vi "Add System.vi"(8 "error in (no error)":errorcluster, 11 "Manager in":refnum<class "Manager.lvclass">) -> (0 "error out":errorcluster, 3 "Manager out":refnum<class "Manager.lvclass">)   [LabVIEW 2013, in "Manager.lvlib" / "Manager.lvclass"]
uses:
  Manager.lvclass
  PluginInterface/Actor Framework.lvlibp/Actor/Actor.lvclass
  Manager Messages/Update SubPanel Msg/Update SubPanel Msg.lvclass
  <vilib>/Utility/LVLibp/NI_PackedLibraryUtility.lvlib
  PluginInterface/PluginInterface.lvlibp/PluginInterfaceClass/PluginInterface.lvclass
  PluginInterface/Actor Framework.lvlibp/Message Enqueuer/Message Enqueuer.lvclass
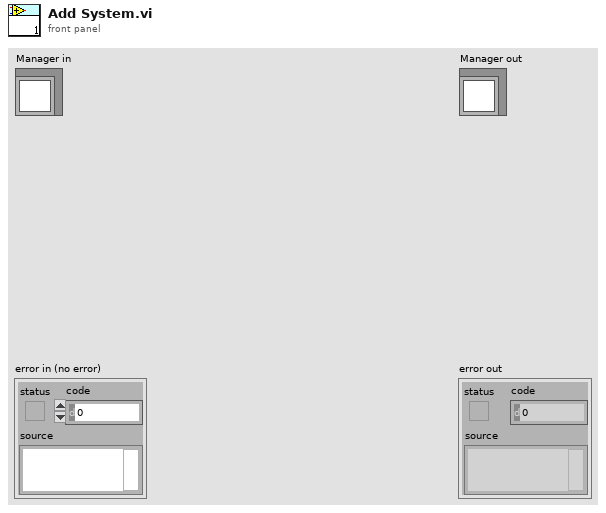
[diagram p1: front panel]
types:
  T1 = cluster{string, "Caller-To-Actor Enqueuer":refnum<class "Message Enqueuer.lvclass">}
  T2 = cluster{"Name":string, "Plugins":cluster{"Name":string, "Plugin":refnum<class "Message Enqueuer.lvclass">}[]}[]
  T3 = cluster{"Name":string, cluster{string, "Caller-To-Actor Enqueuer":refnum<class "Message Enqueuer.lvclass">}[]}
  T4 = cluster{"Name":string, "Plugins":cluster{"Name":string, "Caller-To-Actor Enqueuer":refnum<class "Message Enqueuer.lvclass">}[]}[]
  T5 = cluster{"Name":string, refnum<class "Message Enqueuer.lvclass">[]}
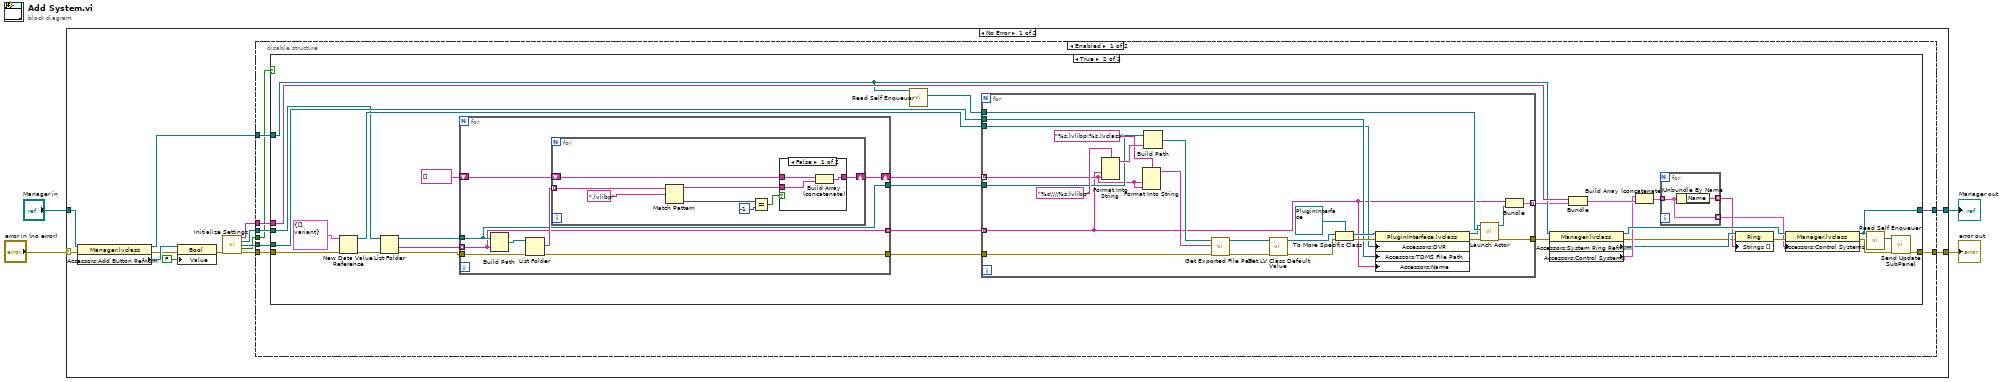
[diagram p0: block diagram]
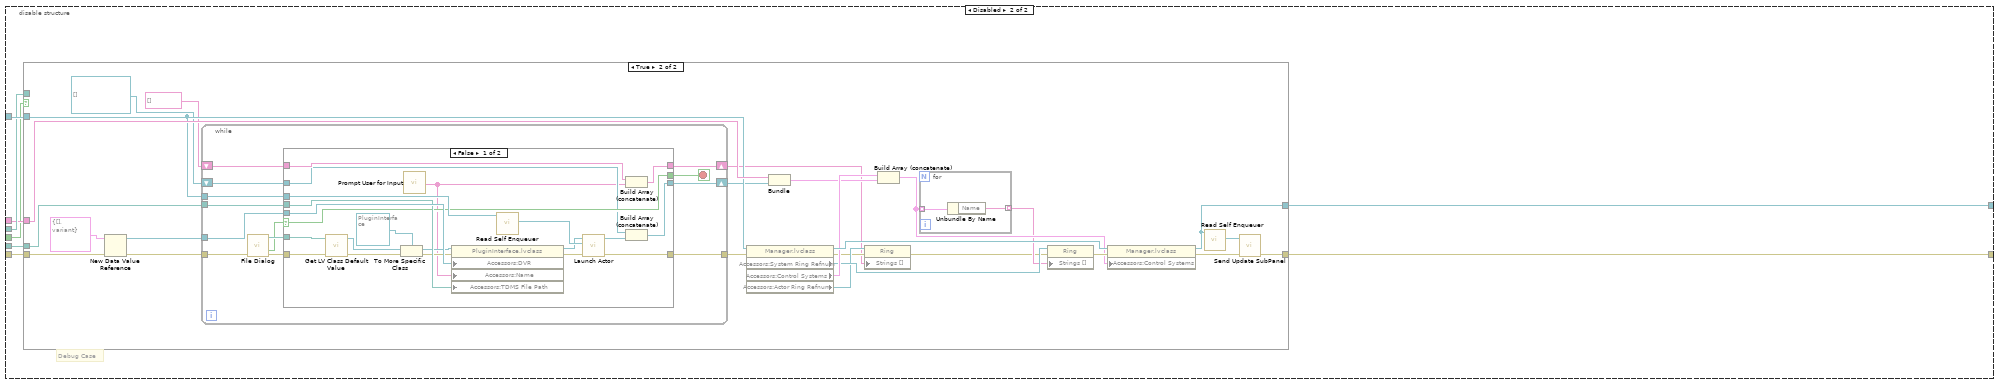
[diagram p4: hidden frame]
diagram:
  n1 = case shown="No Error" "error in (no error)" {
    selector: "error in (no error)" -> [w11 w184]
    tunnel: [w18 w184] -> w3
    tunnel: [w15 w183] -> w1
    tunnel: "Manager in" -> [w9 w183]
    frame No Error {
      n2 = property class="Manager.lvclass"(reference=w9, error in=w11) -> (reference out=w8:refnum<class "Manager.lvclass">, error out=w12:errorcluster, "Accessors:Add Button Refnum"=w14:refnum<vi>)
      n3 = property class="Bool"(reference=w14, error in=w12, "Value"=FALSE ("duplicate session (F)")) -> (error out=w10:errorcluster)  [unwired: 1 out]
      n4 = call "Initialize Settings.vi"("error in (no error)"=w10) -> ("Name"=w6:string, "Plugins Folder 2"=w7:path, "Data Logging Folder 2"=w16:path, "bool"=w5:bool, "error out"=w17:errorcluster)  [unwired: 10 in]
      n5 = disable-structure shown="Enabled" {
        disable-tunnel: [w26 w114] -> w18
        disable-tunnel: w17 -> [w25 w113]
        disable-tunnel: w16 -> [w24 w112]
        disable-tunnel: [w23 w111] -> w15
        disable-tunnel: w8 -> [w22 w110]
        disable-tunnel: w7 -> [w21 w109]
        disable-tunnel: w6 -> [w20 w108]
        disable-tunnel: w5 -> [w19 w107]
        frame Enabled {
          n6 = case shown="True" w19 {
            tunnel: [w28 w55] -> w26
            tunnel: w25 -> [w28 w39]
            tunnel: w24 -> [_ w37]
            tunnel: w21 -> [_ w36]
            tunnel: w22 -> [w27 w41]
            tunnel: w20 -> [_ w50]
            tunnel: [w27 w58] -> w23
            frame False {
            }
            frame True {
              n7 = New Data Value Reference(data value=cluster{string[], "variant":variant} {[], "variant"=variant}, error in=w39) -> (data value reference=w38:refnum<data-value>, error out=w35:errorcluster)
              n8 = List Folder(path=w36, error in=w35) -> (path out=w48:path, folder names=w47:string[], error out=w44:errorcluster)  [unwired: 2 in, 1 out]
              n9 = for {
                tunnel: w47 -> [w85] mode=indexing
                tunnel: w48 -> [w88]
                shift-right: [w89] -> w45
                shift-left: string[] [] -> [w90]
                tunnel: [w88] -> w46
                tunnel: w44 -> [w87]
                tunnel: [w86] -> w43
                tunnel: [w85] -> w33 mode=indexing
                n10 = Build Path(base path=w88, name or relative path=w85) -> (appended path=w92:path)
                n11 = List Folder(path=w92, error in=w87) -> (filenames=w91:string[], error out=w86:errorcluster)  [unwired: 2 in, 2 out]
                n12 = for {
                  tunnel: w91 -> [w97] mode=indexing
                  shift-right: [w98] -> w89
                  shift-left: w90 -> [w99]
                  n13 = Match Pattern(string=w97, regular expression=".lvlibp" ("string")) -> (before substring=w93:string, offset past match=w95:i32)  [unwired: 1 in, 2 out]
                  n14 = Equal?(x=w95, y=-1) -> (x = y?=w100:bool)
                  n15 = case shown="False" w100 {
                    tunnel: w93 -> [w103 _]
                    tunnel: w99 -> [w102 w104]
                    tunnel: [w101 w104] -> w98
                    frame False {
                      n16 = Build Array (concatenate)(w102, w103) -> (w101:string[])
                    }
                    frame True {
                    }
                  }
                }
              }
              n17 = call "Read Self Enqueuer.vi"("Actor"=w41) -> ("Self Enqueuer"=w42:refnum<class "Message Enqueuer.lvclass">)  [unwired: 10 in]
              n18 = for {
                tunnel: w46 -> [w77]
                tunnel: w45 -> [w76] mode=indexing
                tunnel: w43 -> [w75]
                tunnel: [w69] -> w40
                tunnel: w42 -> [w68]
                tunnel: w38 -> [w66]
                tunnel: w37 -> [w67]
                tunnel: w33 -> [w62] mode=indexing
                tunnel: [w61] -> w32 mode=indexing
                n19 = Format Into String(format string="%s\\\\%s.lvlibp", w62, w76) -> (resulting string=w83:string)  [unwired: 2 in, 1 out]
                n20 = Format Into String(format string="%s.lvlibp:%s.lvclass", w76, w76) -> (resulting string=w79:string)  [unwired: 2 in, 1 out]
                n21 = Build Path(base path=w77, name or relative path=w83) -> (appended path=w82:path)
                n22 = call <vilib>:"Get Exported File Path.vi"("error in (no error)"=w75, "qualified name"=w79, "packed library path"=w82) -> ("error out"=w74:errorcluster, "path"=w80:path)  [unwired: 7 in]
                n23 = call <vilib>:"Get LV Class Default Value.vi"("error in (no error)"=w74, "class path"=w80) -> ("error out"=w73:errorcluster, "object"=w78:refnum<class>)  [unwired: 8 in]
                n24 = To More Specific Class(target class=refnum<class "PluginInterface.lvclass"> refnum ("PluginInterface.lvlibp:PluginInterface.lvclass"), reference=w78, error in=w73) -> (specific class reference=w72:refnum<class "PluginInterface.lvclass">, error out=w71:errorcluster)
                n25 = property class="PluginInterface.lvclass"(reference=w72, error in=w71, "Accessors:DVR"=w66, "Accessors:TDMS File Path"=w67, "Accessors:Name"=w62) -> (reference out=w64:refnum<class "PluginInterface.lvclass">, error out=w65:errorcluster)
                n26 = call "Launch Actor.vi"("error in (no error)"=w65, "Actor-to-Caller Enqueuer"=w68, "Actor"=w64) -> ("error out"=w69:errorcluster, "Caller-To-Actor Enqueuer"=w63:refnum<class "Message Enqueuer.lvclass">)  [unwired: 7 in]
                n27 = Bundle(w62, "Caller-To-Actor Enqueuer"=w63) -> (w61:T1)  [unwired: 1 in]
              }
              n28 = property class="Manager.lvclass"(reference=w41, error in=w40) -> (reference out=w59:refnum<class "Manager.lvclass">, error out=w31:errorcluster, "Accessors:System Ring Refnum"=w53:refnum<vi>, "Accessors:Control Systems"=w54:T2)
              n29 = Bundle("Name"=w50, w32) -> (w60:T3)  [unwired: 1 in]
              n30 = Build Array (concatenate)(w54, w60) -> (w30:T4)
              n31 = for {
                tunnel: w30 -> [w105] mode=indexing
                tunnel: [w106] -> w51 mode=indexing
                tunnel: [w105] -> w29 mode=indexing
                n32 = Unbundle By Name(w105) -> ("Name"=w106:string)
              }
              n33 = property class="Ring"(reference=w53, error in=w31, "Strings []"=w51) -> (error out=w52:errorcluster)  [unwired: 1 out]
              n34 = property class="Manager.lvclass"(reference=w59, error in=w52, "Accessors:Control Systems"=w29) -> (reference out=w58:refnum<class "Manager.lvclass">, error out=w56:errorcluster)
              n35 = call "Read Self Enqueuer.vi"("Actor"=w58) -> ("Self Enqueuer"=w57:refnum<class "Message Enqueuer.lvclass">)  [unwired: 10 in]
              n36 = call "Send Update SubPanel.vi"("error in (no error)"=w56, "Message Enqueuer"=w57) -> ("error out"=w55:errorcluster)  [unwired: 8 in, 1 out]
            }
          }
        }
        frame Disabled {
          # "Debug Case"
          n37 = case shown="True" w107 {
            tunnel: [w116 w138] -> w114
            tunnel: w113 -> [w116 w126]
            tunnel: w112 -> [_ w124]
            tunnel: w109 -> [_ _]
            tunnel: w110 -> [w115 w131]
            tunnel: w108 -> [_ w132]
            tunnel: [w115 w141] -> w111
            frame False {
            }
            frame True {
              n38 = New Data Value Reference(data value=cluster{string[], "variant":variant} {[], "variant"=variant}, error in=w126) -> (data value reference=w125:refnum<data-value>, error out=w122:errorcluster)
              n39 = while {
                tunnel: w131 -> [w155]
                tunnel: [w154] -> w127
                tunnel: w125 -> [w153]
                tunnel: w124 -> [w152]
                tunnel: w122 -> [w151]
                shift-right: [w144] -> w117
                shift-left: string[] [] -> [w143]
                shift-right: [w145] -> w118
                shift-left: refnum<class "Message Enqueuer.lvclass">[] [] -> [w146]
                stop <- w147 stop-if-true
                n40 = call "File Dialog"("error in"=w151) -> ("selected path"=w149:path, "cancelled"=w148:bool, "error out"=w150:errorcluster)  [unwired: 11 in, 1 out]
                n41 = case shown="False" w148 {
                  selector: w148 -> [w162 w180]
                  tunnel: w155 -> [w175 _]
                  tunnel: [w174 w179] -> w154
                  tunnel: w153 -> [w173 _]
                  tunnel: w152 -> [w172 _]
                  tunnel: w150 -> [w166 w179]
                  tunnel: w149 -> [w165 _]
                  tunnel: [w158 w178] -> w145
                  tunnel: [w157 w177] -> w144
                  tunnel: [w162 w180] -> w147
                  tunnel: w146 -> [w160 w178]
                  tunnel: w143 -> [w161 w177]
                  frame False {
                    n42 = call <vilib>:"Get LV Class Default Value.vi"("error in (no error)"=w166, "class path"=w165) -> ("error out"=w170:errorcluster, "object"=w171:refnum<class>)  [unwired: 8 in]
                    n43 = To More Specific Class(target class=refnum<class "PluginInterface.lvclass"> refnum ("PluginInterface.lvlibp:PluginInterface.lvclass"), reference=w171, error in=w170) -> (specific class reference=w169:refnum<class "PluginInterface.lvclass">, error out=w168:errorcluster)
                    n44 = call "Prompt User for Input"() -> ("name"=w156:string)  [unwired: 17 in, 2 out]
                    n45 = property class="PluginInterface.lvclass"(reference=w169, error in=w168, "Accessors:DVR"=w173, "Accessors:Name"=w156, "Accessors:TDMS File Path"=w172) -> (reference out=w164:refnum<class "PluginInterface.lvclass">, error out=w163:errorcluster)
                    n46 = call "Read Self Enqueuer.vi"("Actor"=w175) -> ("Self Enqueuer"=w176:refnum<class "Message Enqueuer.lvclass">)  [unwired: 10 in]
                    n47 = call "Launch Actor.vi"("error in (no error)"=w163, "Actor-to-Caller Enqueuer"=w176, "Actor"=w164) -> ("error out"=w174:errorcluster, "Caller-To-Actor Enqueuer"=w159:refnum<class "Message Enqueuer.lvclass">)  [unwired: 7 in]
                    n48 = Build Array (concatenate)(w161, w156) -> (w157:string[])
                    n49 = Build Array (concatenate)(w160, w159) -> (w158:refnum<class "Message Enqueuer.lvclass">[])
                  }
                  frame True {
                  }
                }
              }
              n50 = property class="Manager.lvclass"(reference=w131, error in=w127) -> (reference out=w142:refnum<class "Manager.lvclass">, error out=w129:errorcluster, "Accessors:System Ring Refnum"=w136:refnum<vi>, "Accessors:Control Systems"=w137:T2, "Accessors:Actor Ring Refnum"=w130:refnum<vi>)
              n51 = Bundle("Name"=w132, w118) -> (w121:T5)  [unwired: 1 in]
              n52 = property class="Ring"(reference=w130, error in=w129, "Strings []"=w117) -> (error out=w128:errorcluster)  [unwired: 1 out]
              n53 = Build Array (concatenate)(w137, w121) -> (w134:T2)
              n54 = for {
                tunnel: w134 -> [w182] mode=indexing
                tunnel: [w181] -> w133 mode=indexing
                n55 = Unbundle By Name(w182) -> ("Name"=w181:string)
              }
              n56 = property class="Ring"(reference=w136, error in=w128, "Strings []"=w133) -> (error out=w135:errorcluster)  [unwired: 1 out]
              n57 = property class="Manager.lvclass"(reference=w142, error in=w135, "Accessors:Control Systems"=w134) -> (reference out=w141:refnum<class "Manager.lvclass">, error out=w139:errorcluster)
              n58 = call "Read Self Enqueuer.vi"("Actor"=w141) -> ("Self Enqueuer"=w140:refnum<class "Message Enqueuer.lvclass">)  [unwired: 10 in]
              n59 = call "Send Update SubPanel.vi"("error in (no error)"=w139, "Message Enqueuer"=w140) -> ("error out"=w138:errorcluster)  [unwired: 8 in, 1 out]
            }
          }
        }
      }
    }
    frame Error {
    }
  }
  "error out" <- w3
  "Manager out" <- w1
